vi "WakeOnLAN.vi"(10 "Mac Address":string="\u0000\u0018‹\u001dš#", 11 "IP of the computer to control":string="192.168.126.44") -> ()   [LabVIEW 2012]
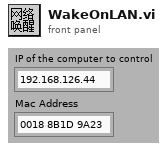
[diagram p1: front panel]
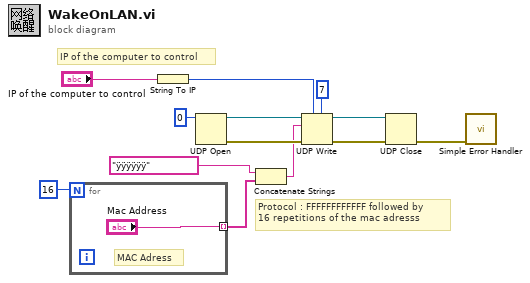
[diagram p0: block diagram]
diagram:
  # "IP of the computer to control"
  # "Protocol : FFFFFFFFFFFF followed by\n16 repetitions of the mac adresss"
  n1 = for {
    N: 16 -> [_]
    tunnel: ["Mac Address"] -> w2 mode=indexing
    # "MAC Adress"
  }
  n2 = String To IP(1:"IP of the computer to control") -> (0:w11:u32)
  n3 = UDP Open(11:u16 0 ("port")) -> (port=w9:refnum<k16>, 0:w7:errorcluster)  [unwired: 4 in, 1 out]
  n4 = Concatenate Strings("ÿÿÿÿÿÿ", w2) -> (w1:string)
  n5 = UDP Write(address=w11, port or service name=u16 7, connection ID=w9, data in=w1, 8:w7) -> (error out=w6:errorcluster, 3:w8:refnum<k16>)  [unwired: 1 in]
  n6 = UDP Close(connection ID=w8, 8:w6) -> (error out=w5:errorcluster)  [unwired: 1 out]
  n7 = call <vilib>:"Simple Error Handler.vi"("error in (no error)"=w5) -> ()  [unwired: 4 in, 5 out]
